vi "Validate Parameters.vi"(8 "error in":errorcluster, 11 "path of type":path) -> (0 "error out":errorcluster, 2 "parameters with invalid type":string[](array[string]), 3 "parameter names":string[](array[string]))   [LabVIEW 2021, in "NI Measurement Plug-In SDK.lvlib"]
uses:
  NI Measurement Plug-In SDK.lvlib
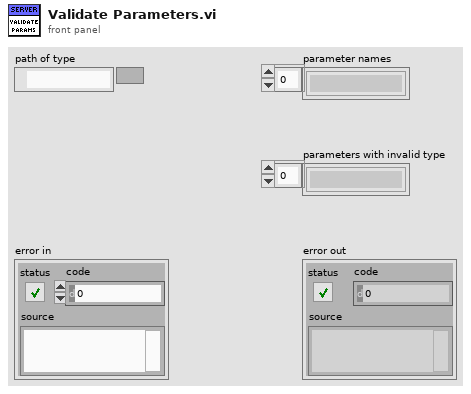
[diagram p1: front panel]
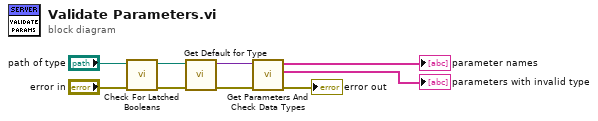
[diagram p0: block diagram]
diagram:
  n1 = call "Check For Latched Booleans.vi"("error in"="error in", "path of type"="path of type") -> ("error out"=w7:errorcluster, "path of type out"=w6:path)  [unwired: 8 in]
  n2 = call "Get Default for Type.vi"("error in"=w7, "path of type"=w6) -> ("error out"=w3:errorcluster, "default for type"=w2:variant)  [unwired: 8 in]
  n3 = call "Get Parameters And Check Data Types.vi"("error in"=w3, "variant"=w2) -> ("error out"=→"error out":errorcluster, "parameters with invalid type"=→"parameters with invalid type":string[], "parameter names"=→"parameter names":string[])  [unwired: 7 in]
